vi "UI_List.vi"() -> ()   [LabVIEW 2016]
uses:
  PanelSplitToolkit/QueueManager.llb/Remove.vi
  <vilib>/Utility/error.llb/DialogType.ctl
  PanelSplitToolkit/QueueManager.llb/Valid?.vi
  PanelSplitToolkit/QueueManager.llb/Insert.vi
  PanelSplitToolkit/QueueManager.llb/Destroy.vi
  <vilib>/Platform/TimedLoop/XDataNode/XDataNode.xnode
  <vilib>/Platform/TimedLoop/XDataNode/nitl_modes.ctl
  <vilib>/Platform/TimedLoop/XDataNode/XDNodeRunTimeDep.lvlib
  <vilib>/Platform/TimedLoop/XDataNode/wakeup.ctl
  <vilib>/Platform/TimedLoop/XDataNode/timing_clust.ctl
  SelectPoint2011/SelectPointObj/SelectPointObj.lvclass
  SelectPoint2011/ManualSelectPoint/ManualSelectPoint.lvclass
  <vilib>/Utility/miscctls.llb/LVRowAndColumnTypeDef.ctl
  PanelSplitToolkit/QueueManager.llb/CreatQueue.vi
panel:
  in  "ID":string caption="请输入产品编号:"
  in  "Caller":string
  in  "Pause":bool
  in  "Stop":bool
  in  "手动":bool
  in  "开始":bool
  in  "多列列表框":i32(listbox)
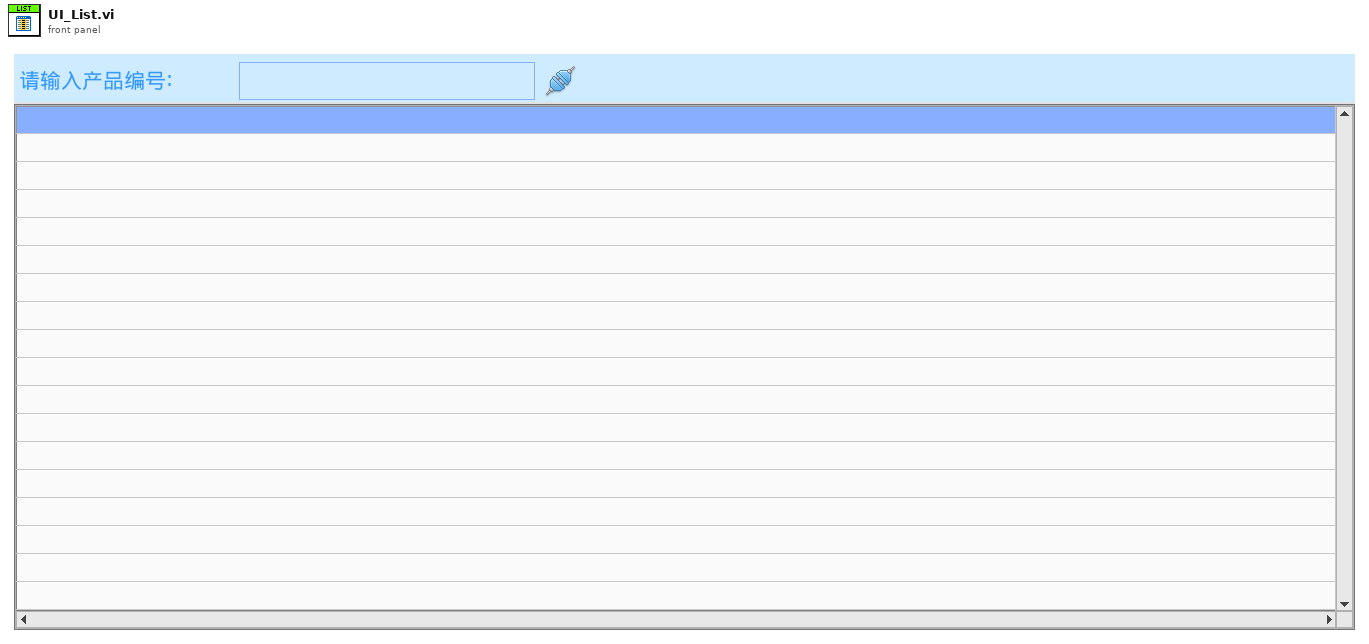
[diagram p1: front panel]
types:
  T1 = cluster{"error":errorcluster, "Event":string, "Data":variant, "Q_Local":string, "SelectPointClass":refnum<class "SelectPointObj.lvclass">, "Q_Caller":string, "ListRef":refnum<vi>}
  T2 = typedef "XDNodeRunTimeDep.lvlib/timing_clust.ctl" = cluster{"Expected End [f-1]":u64, "Actual End [f-1]":u64, "Finished Late? [f-1]":bool, "Expected End [i-1]":u64, "Actual End [i-1]":u64, "Finished Late? [i-1]":bool, "Expected Start [i]":u64, "Actual Start [i]":u64, "Expected Start [f]":u64, "Actual Start [f]":u64, "Source Name":string, "Structure Name":string, "Period":i64, "Deadline":i64, "Offset":i64, "Start":i64, "Priority":i32, "Timeout":i32, "Mode":T3, "Wakeup Reason":T4, "Error":errorcluster, "Source Type":string, "Secondary Source Type":string, "Global End Time":u64, "Global Start Time":u64, "Frame Duration":u64, "Iteration Duration":u64, "Assigned CPU":i32, "I/O Scan Engine Mode":u32}
  T3 = typedef "XDNodeRunTimeDep.lvlib/nitl_modes.ctl" = enum32{"No Change", "Process missed periods, maintain original phase", "Discard missed periods, maintain original phase", "Process missed periods, ignore original phase", "Discard missed periods, ignore original phase"}
  T4 = typedef "XDNodeRunTimeDep.lvlib/wakeup.ctl" = enum32{"Normal", "Aborted", "Asynchronous wakeup", "Timing source error", "Timed loop error", "Timeout"}
  T5 = cluster{"Font Name":string, "Size":u16, "Bold":bool, "Italic":bool, "Underline":bool, "Strikeout":bool, "color":u32}
  T6 = typedef "LVRowAndColumnTypeDef.ctl" = cluster{"Row":i32, "Column":i32}
  T7 = typedef "DialogType.ctl" = u16
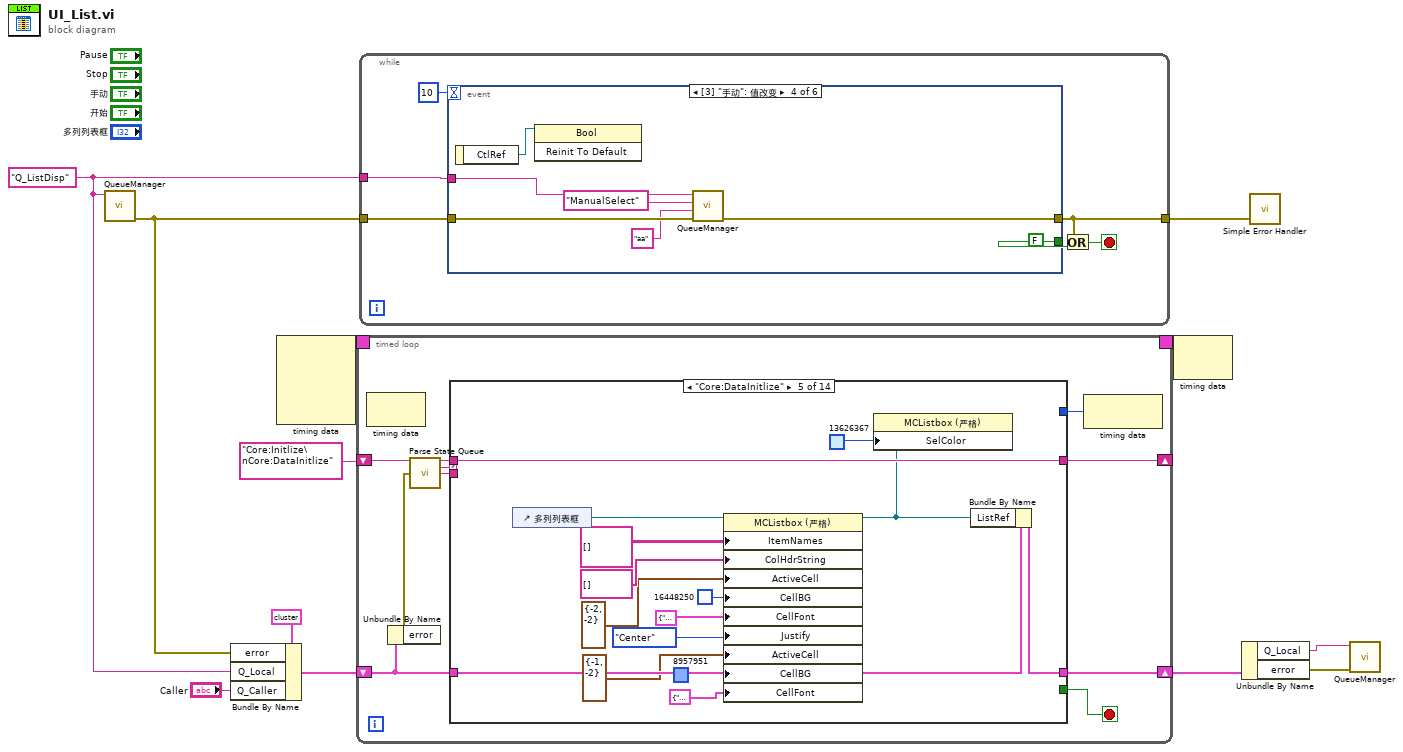
[diagram p0: block diagram]
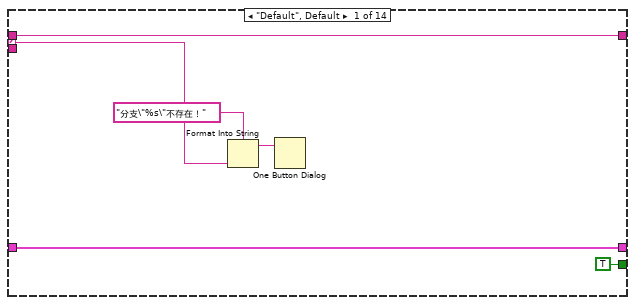
[diagram p2: hidden frame]
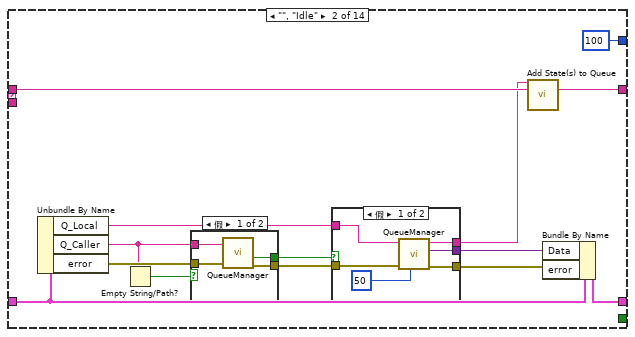
[diagram p3: hidden frame]
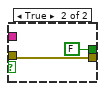
[diagram p4: hidden frame]
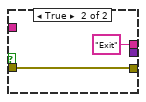
[diagram p5: hidden frame]
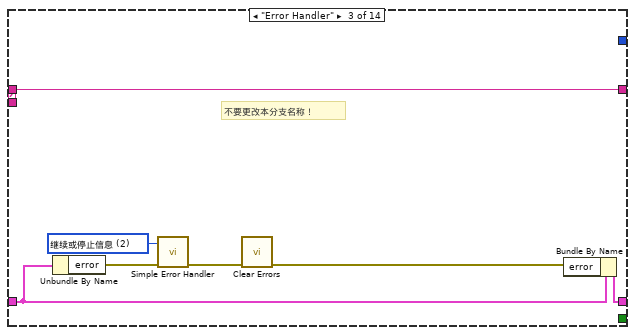
[diagram p6: hidden frame]
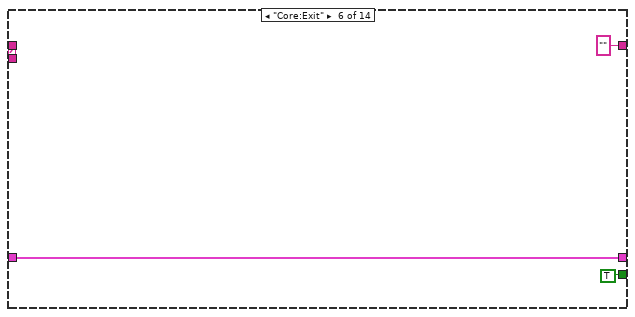
[diagram p8: hidden frame]
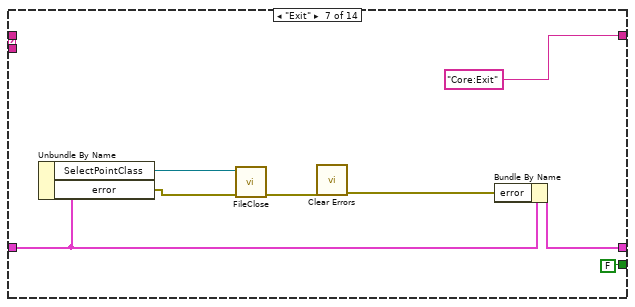
[diagram p9: hidden frame]
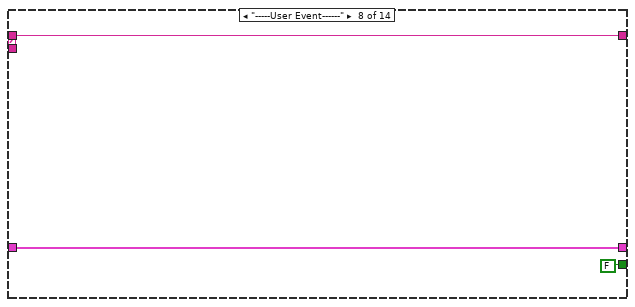
[diagram p10: hidden frame]
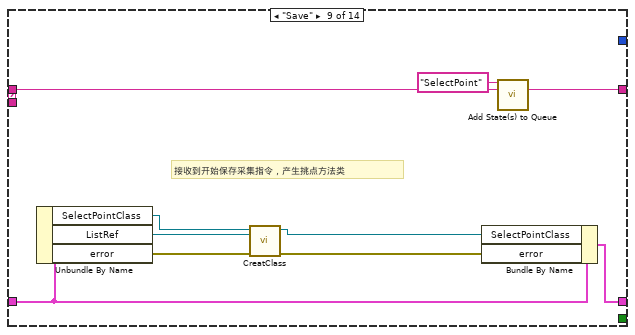
[diagram p11: hidden frame]
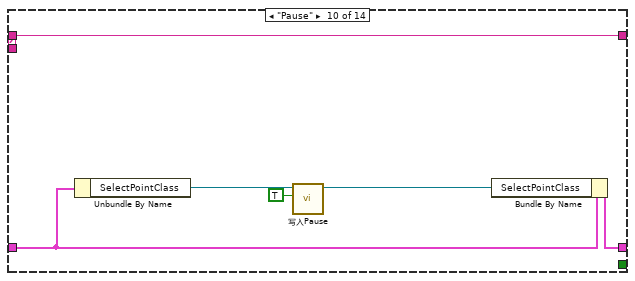
[diagram p12: hidden frame]
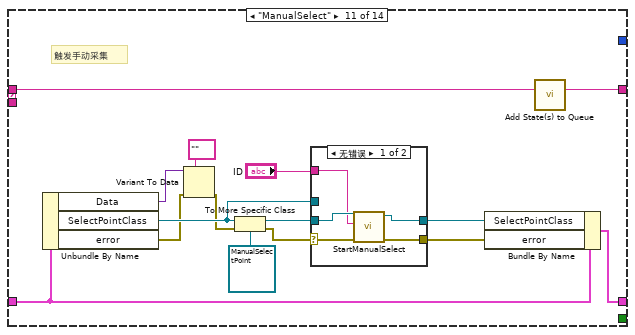
[diagram p13: hidden frame]
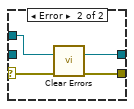
[diagram p14: hidden frame]
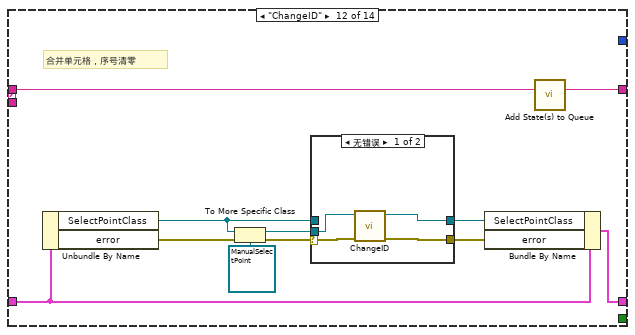
[diagram p15: hidden frame]
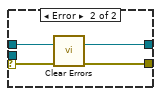
[diagram p16: hidden frame]
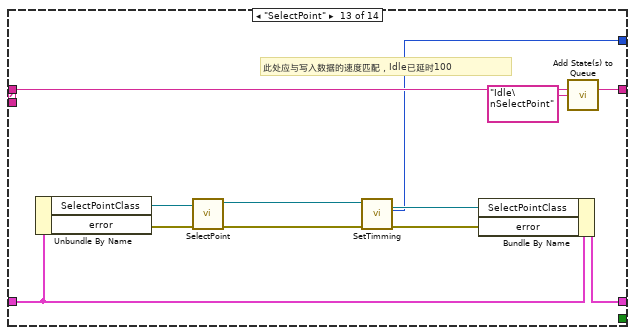
[diagram p17: hidden frame]
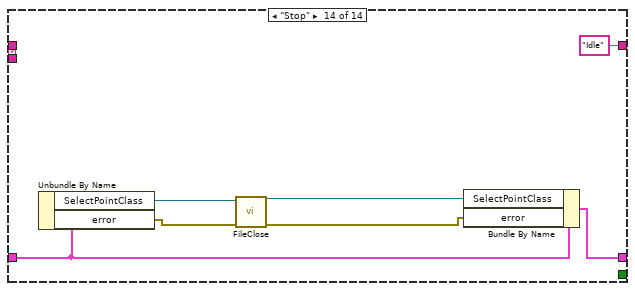
[diagram p18: hidden frame]
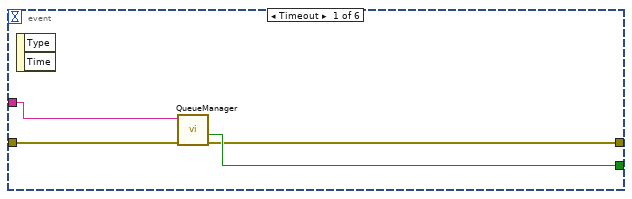
[diagram p19: hidden frame]
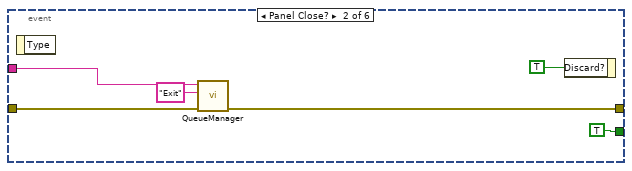
[diagram p20: hidden frame]
diagram:
  w6 = "Q_ListDisp" ("QueueName")
  n1 = call-poly "QueueManager.vi"("QueueName"=w6) -> ("error out"=w4:errorcluster)  [unwired: 9 in, 1 out]
  n2 = Bundle By Name(cluster=T1 {"error"={"status"=FALSE, "code"=0, "source"=""}, "Event"="", "Data"=variant, "Q_Local"="", "SelectPointClass"=refnum, "Q_Caller"="", "ListRef"=refnum} ("TmpData"), "error"=w4, "Q_Local"=w6, "Q_Caller"="Caller") -> (w7:T1)
  n3 = node-c288() -> (w3:T2)  [unwired: 4 in]
  n4 = timed-loop {
    shift-right: [w15] -> w10
    shift-left: w7 -> [w16]
    shift-right: [w14] -> _
    shift-left: "Core:Initlize\nCore:DataInitlize" -> [w22]
    timing: w3 -> [_]
    timing-out: [_] -> w2
    stop <- w18 stop-if-true
    n5 = node-c288() -> ()  [unwired: 1 in, 1 out]
    n6 = Unbundle By Name(w16) -> ("error"=w17:errorcluster)
    n7 = call "Parse State Queue.vi"("State Queue"=w22, "Error In (no error)"=w17) -> ("Remaining States"=w21:string, "Current State"=w20:string, "Arguments"=w19:string)  [unwired: 10 in, 1 out]
    n8 = case shown="\"Core:DataInitlize\"" w20 {
      selector: w20 -> [w30 _ _ _ _ _ _ _ _ _ _ _ _ _]
      tunnel: w21 -> [w31 w43 w67 w69 w84 _ _ w96 w103 w114 w129 w148 w167 _]
      tunnel: w19 -> [_ _ _ _ _ _ _ _ _ _ _ _ _ _]
      tunnel: [TRUE _ _ _ _ TRUE FALSE FALSE _ _ _ _ _ _] -> w18
      tunnel: w16 -> [w32 w42 w63 w68 w83 w86 w91 w97 w106 w110 w127 w146 w165 w171]
      tunnel: [w32 w45 w62 w68 w82 w86 w90 w97 w104 w109 w126 w145 w164 w170] -> w15
      tunnel: [w31 w41 w67 w69 w84 "" ("Remaining States") "Core:Exit" ("Remaining States") w96 w102 w114 w128 w147 w166 "Idle" ("States Out")] -> w14
      tunnel: [_ i64 100 ("周期") _ _ _ _ _ _ _ _ _ _ w162 _] -> w13
      frame "Default", Default {
        n9 = Format Into String(format string="分支\"%s\"不存在！" ("格式字符串"), w30) -> (resulting string=w29:string)  [unwired: 2 in, 1 out]
        n10 = One Button Dialog(message=w29) -> ()  [unwired: 1 in, 1 out]
      }
      frame "", "Idle" {
        n11 = Unbundle By Name(w42) -> ("Q_Local"=w39:string, "Q_Caller"=w35:string, "error"=w38:errorcluster)
        n12 = Empty String/Path?(string/path=w35) -> (empty?=w34:bool)
        n13 = case shown="假" w34 {
          tunnel: w38 -> [w50 w51]
          tunnel: [w49 w51] -> w37
          tunnel: [w48 FALSE ("Not Exist?")] -> w36
          tunnel: w35 -> [w47 _]
          frame False {
            n14 = call-poly "QueueManager.vi"("error in (no error)"=w50, "Queue Name(unamed)"=w47) -> ("error out"=w49:errorcluster, "Not Exist?"=w48:bool)  [unwired: 8 in]
          }
          frame True {
          }
        }
        n15 = case shown="假" w36 {
          tunnel: [w58 w59] -> w46
          tunnel: [w57 _] -> w44
          tunnel: [w56 "Exit" ("Event")] -> w33
          tunnel: w39 -> [w54 _]
          tunnel: w37 -> [w53 w59]
          frame False {
            n16 = call-poly "QueueManager.vi"("Time out(-1)"=50, "error in (no error)"=w53, "Queue Name"=w54) -> ("error out"=w58:errorcluster, "Data"=w57:variant, "Event"=w56:string)  [unwired: 5 in, 1 out]
          }
          frame True {
          }
        }
        n17 = call "Add State(s) to Queue.vi"("State(s) in Front (\"\")"=w33, "State(s) in (\"\")"=w43) -> ("States Out"=w41:string)  [unwired: 13 in]
        n18 = Bundle By Name(cluster=w42, "Data"=w44, "error"=w46) -> (w45:T1)
      }
      frame "Error Handler" {
        w61 = T7 2 items=["无对话框", "确定信息", "继续或停止信息", "确定信息＋警告", "继续/停止+警告"] ("type of dialog (OK msg:1)")
        # "不要更改本分支名称！"
        n19 = Unbundle By Name(w63) -> ("error"=w64:errorcluster)
        n20 = call <vilib>:"Simple Error Handler.vi"("type of dialog (OK msg:1)"=w61, "error in (no error)"=w64) -> ("error out"=w65:errorcluster)  [unwired: 3 in, 4 out]
        n21 = call <vilib>:"Clear Errors.vi"("error in (no error)"=w65) -> ("error out"=w66:errorcluster)  [unwired: 5 in, 1 out]
        n22 = Bundle By Name(cluster=w63, "error"=w66) -> (w62:T1)
      }
      frame "Core:Initlize" {
      }
      frame "Core:DataInitlize" {
        n23 = control-ref of="多列列表框"() -> (w81:refnum<vi>)
        n24 = property class="MCListbox (严格)"(reference=w81, "ItemNames"=string[][] [] ("项名"), "ColHdrString"=string[] [] ("列首字符串[]"), "ActiveCell"=T6 {"Row"=-2, "Column"=-2} ("活动单元格:活动单元格"), "CellBG"=u32 16448250, "CellFont"=T5 {"Font Name"="Tahoma", "Size"=24, "Bold"=FALSE, "Italic"=FALSE, "Underline"=FALSE, "Strikeout"=FALSE, "color"=3381759} ("Active Cell:Cell Font"), "Justify"=enum16{"Left", "Center", "Right"}."Center" ("活动单元格:单元格对齐"), "ActiveCell"=T6 {"Row"=-1, "Column"=-2} ("活动单元格:活动单元格"), "CellBG"=u32 8957951, "CellFont"=T5 {"Font Name"="Tahoma", "Size"=24, "Bold"=FALSE, "Italic"=FALSE, "Underline"=FALSE, "Strikeout"=FALSE, "color"=16448250} ("Active Cell:Cell Font")) -> (reference out=w71:refnum<vi>)  [unwired: 1 in, 1 out]
        n25 = property class="MCListbox (严格)"(reference=w71, "SelColor"=u32 13626367) -> ()  [unwired: 1 in, 2 out]
        n26 = Bundle By Name(cluster=w83, "ListRef"=w71) -> (w82:T1)
      }
      frame "Core:Exit" {
      }
      frame "Exit" {
        n27 = Unbundle By Name(w91) -> ("SelectPointClass"=w93:refnum<class "SelectPointObj.lvclass">, "error"=w92:errorcluster)
        n28 = call-dynamic "FileClose.vi"("error in (no error)"=w92, "SelectPointObj 输入"=w93) -> ("error out"=w89:errorcluster)  [unwired: 8 in, 1 out]
        n29 = call <vilib>:"Clear Errors.vi"("error in (no error)"=w89) -> ("error out"=w88:errorcluster)  [unwired: 5 in, 1 out]
        n30 = Bundle By Name(cluster=w91, "error"=w88) -> (w90:T1)
      }
      frame "-----User Event------" {
      }
      frame "Save" {
        # "接收到开始保存采集指令，产生挑点方法类"
        n31 = Unbundle By Name(w106) -> ("SelectPointClass"=w99:refnum<class "SelectPointObj.lvclass">, "ListRef"=w100:refnum<vi>, "error"=w108:errorcluster)
        n32 = call "CreatClass.vi"("error in"=w108, "ListRef"=w100, "SelectPointObj"=w99) -> ("error out"=w107:errorcluster, "SelectPointObj.lvclass"=w105:refnum<class "SelectPointObj.lvclass">)  [unwired: 7 in]
        n33 = Bundle By Name(cluster=w106, "SelectPointClass"=w105, "error"=w107) -> (w104:T1)
        n34 = call "Add State(s) to Queue.vi"("State(s) in Front (\"\")"="SelectPoint" ("State(s) in Front (\"\")"), "State(s) in (\"\")"=w103) -> ("States Out"=w102:string)  [unwired: 13 in]
      }
      frame "Pause" {
        n35 = Unbundle By Name(w110) -> ("SelectPointClass"=w113:refnum<class "SelectPointObj.lvclass">)
        n36 = call-dynamic "写入Pause.vi"("Pause?"=TRUE, "SelectPointObj输入"=w113) -> ("SelectPointObj输出"=w111:refnum<class "SelectPointObj.lvclass">)  [unwired: 8 in, 1 out]
        n37 = Bundle By Name(cluster=w110, "SelectPointClass"=w111) -> (w109:T1)
      }
      frame "ManualSelect" {
        # "触发手动采集"
        n38 = Unbundle By Name(w127) -> ("Data"=w119:variant, "SelectPointClass"=w120:refnum<class "SelectPointObj.lvclass">, "error"=w118:errorcluster)
        n39 = Variant To Data(error in=w118, type="", Variant=w119) -> (error out=w117:errorcluster)  [unwired: 1 out]
        n40 = To More Specific Class(target class=refnum<class "ManualSelectPoint.lvclass"> refnum ("ManualSelectPoint.lvclass"), reference=w120, error in=w117) -> (specific class reference=w123:refnum<class "ManualSelectPoint.lvclass">, error out=w124:errorcluster)
        n41 = case shown="无错误" w124 {
          selector: w124 -> [w133 w136]
          tunnel: w123 -> [w134 _]
          tunnel: [w132 w135] -> w122
          tunnel: [w131 w137] -> w121
          tunnel: w120 -> [_ w137]
          tunnel: "ID" -> [w130 _]
          frame No Error {
            n42 = call "StartManualSelect.vi"("error in"=w133, "ProductID"=w130, "ManualSelectPoint 输入"=w134) -> ("error out"=w132:errorcluster, "ManualSelectPoint 输出"=w131:refnum<class "ManualSelectPoint.lvclass">)  [unwired: 7 in]
          }
          frame Error {
            n43 = call <vilib>:"Clear Errors.vi"("error in (no error)"=w136) -> ("error out"=w135:errorcluster)  [unwired: 5 in, 1 out]
          }
        }
        n44 = Bundle By Name(cluster=w127, "SelectPointClass"=w121, "error"=w122) -> (w126:T1)
        n45 = call "Add State(s) to Queue.vi"("State(s) in (\"\")"=w129) -> ("States Out"=w128:string)  [unwired: 14 in]
      }
      frame "ChangeID" {
        # "合并单元格，序号清零"
        n46 = Unbundle By Name(w146) -> ("SelectPointClass"=w139:refnum<class "SelectPointObj.lvclass">, "error"=w138:errorcluster)
        n47 = To More Specific Class(target class=refnum<class "ManualSelectPoint.lvclass"> refnum ("ManualSelectPoint.lvclass"), reference=w139, error in=w138) -> (specific class reference=w142:refnum<class "ManualSelectPoint.lvclass">, error out=w143:errorcluster)
        n48 = case shown="无错误" w143 {
          selector: w143 -> [w150 w154]
          tunnel: w142 -> [w152 _]
          tunnel: [w149 w153] -> w141
          tunnel: [w151 w155] -> w140
          tunnel: w139 -> [_ w155]
          frame No Error {
            n49 = call "ChangeID.vi"("error in"=w150, "ManualSelectPoint 输入"=w152) -> ("error out"=w149:errorcluster, "ManualSelectPoint 输出"=w151:refnum<class "ManualSelectPoint.lvclass">)  [unwired: 8 in]
          }
          frame Error {
            n50 = call <vilib>:"Clear Errors.vi"("error in (no error)"=w154) -> ("error out"=w153:errorcluster)  [unwired: 5 in, 1 out]
          }
        }
        n51 = Bundle By Name(cluster=w146, "SelectPointClass"=w140, "error"=w141) -> (w145:T1)
        n52 = call "Add State(s) to Queue.vi"("State(s) in (\"\")"=w148) -> ("States Out"=w147:string)  [unwired: 14 in]
      }
      frame "SelectPoint" {
        # "此处应与写入数据的速度匹配，Idle已延时100"
        n53 = Unbundle By Name(w165) -> ("SelectPointClass"=w159:refnum<class "SelectPointObj.lvclass">, "error"=w158:errorcluster)
        n54 = call-dynamic "SelectPoint.vi"("error in"=w158, "SelectPointObj 输入"=w159) -> ("error out"=w157:errorcluster, "SelectPointObj 输出"=w156:refnum<class "SelectPointObj.lvclass">)  [unwired: 8 in]
        n55 = call-dynamic "SetTimming.vi"("error in (no error)"=w157, "SelectPointObj 输入"=w156) -> ("error out"=w161:errorcluster, "dt"=w162:i64, "SelectPointObj 输出"=w163:refnum<class "SelectPointObj.lvclass">)  [unwired: 7 in]
        n56 = Bundle By Name(cluster=w165, "SelectPointClass"=w163, "error"=w161) -> (w164:T1)
        n57 = call "Add State(s) to Queue.vi"("State(s) in (\"\")"=w167, "State(s) at Back (\"\")"="Idle\nSelectPoint" ("State(s) at Back (\"\")")) -> ("States Out"=w166:string)  [unwired: 13 in]
      }
      frame "Stop" {
        n58 = Unbundle By Name(w171) -> ("SelectPointClass"=w173:refnum<class "SelectPointObj.lvclass">, "error"=w168:errorcluster)
        n59 = call-dynamic "FileClose.vi"("error in (no error)"=w168, "SelectPointObj 输入"=w173) -> ("error out"=w169:errorcluster, "SelectPointObj 输出"=w172:refnum<class "SelectPointObj.lvclass">)  [unwired: 8 in]
        n60 = Bundle By Name(cluster=w171, "SelectPointClass"=w172, "error"=w169) -> (w170:T1)
      }
    }
    n61 = node-c288(w13) -> ()  [unwired: 1 out]
  }
  n62 = while {
    tunnel: w4 -> [w179]
    tunnel: w6 -> [w180]
    tunnel: [w176] -> w9
    stop <- w177 stop-if-true
    n63 = event shown="[3] \"手动\": 值改变" {
      selector: _ -> [_ _ _ _ _ _]
      dyn-events: _ -> [_ _ _ _ _ _]
      timeout: 10 -> [_ _ _ _ _ _]
      tunnel: [w182 TRUE FALSE FALSE FALSE FALSE] -> w178
      tunnel: w180 -> [w184 w189 w195 w202 w208 w214]
      tunnel: w179 -> [w183 w188 w194 w201 w207 w213]
      tunnel: [w181 w187 w193 w200 w206 w212] -> w176
      event Timeout {
        n64 = event-data() -> ()  [unwired: 1 in, 2 out]
        n65 = call-poly "QueueManager.vi"("error in (no error)"=w183, "Queue Name(unamed)"=w184) -> ("error out"=w181:errorcluster, "Not Exist?"=w182:bool)  [unwired: 8 in]
      }
      event Panel Close? {
        n66 = event-data() -> ()  [unwired: 1 in, 1 out]
        n67 = call-poly "QueueManager.vi"("error in"=w188, "Event"="Exit", "QueueName"=w189) -> ("error out"=w187:errorcluster)  [unwired: 7 in, 1 out]
        n68 = event-data("Discard?"=TRUE ("放弃？")) -> ()  [unwired: 1 in, 1 out]
      }
      event "开始": Value Change {
        (unwired) TRUE ("放弃？")
        n69 = event-data() -> ("CtlRef"=w191:refnum<vi>)  [unwired: 1 in]
        n70 = invoke class="Bool" method="Reinit To Default"(reference=w191) -> ()  [unwired: 2 in, 3 out]
        n71 = call-poly "QueueManager.vi"("error in"=w194, "Event"="Save", "QueueName"=w195) -> ("error out"=w193:errorcluster)  [unwired: 7 in, 1 out]
      }
      event "手动": Value Change {
        n72 = event-data() -> ("CtlRef"=w198:refnum<vi>)  [unwired: 1 in]
        n73 = invoke class="Bool" method="Reinit To Default"(reference=w198) -> ()  [unwired: 2 in, 3 out]
        n74 = call-poly "QueueManager.vi"("error in"=w201, "Data"="aa", "Event"="ManualSelect", "QueueName"=w202) -> ("error out"=w200:errorcluster)  [unwired: 6 in, 1 out]
      }
      event "Stop": Value Change {
        (unwired) TRUE ("放弃？")
        n75 = event-data() -> ("CtlRef"=w204:refnum<vi>)  [unwired: 1 in]
        n76 = invoke class="Bool" method="Reinit To Default"(reference=w204) -> ()  [unwired: 2 in, 3 out]
        n77 = call-poly "QueueManager.vi"("error in"=w207, "Event"="Stop", "QueueName"=w208) -> ("error out"=w206:errorcluster)  [unwired: 7 in, 1 out]
      }
      event "Pause": Value Change {
        (unwired) TRUE ("放弃？")
        n78 = event-data() -> ("CtlRef"=w210:refnum<vi>)  [unwired: 1 in]
        n79 = invoke class="Bool" method="Reinit To Default"(reference=w210) -> ()  [unwired: 2 in, 3 out]
        n80 = call-poly "QueueManager.vi"("error in"=w213, "Event"="Pause", "QueueName"=w214) -> ("error out"=w212:errorcluster)  [unwired: 7 in, 1 out]
      }
    }
    n81 = Or(x=w176, y=w178) -> (x .or. y?=w177:bool)
  }
  n82 = node-c288(w2) -> ()  [unwired: 1 out]
  n83 = Unbundle By Name(w10) -> ("Q_Local"=w5:string, "error"=w11:errorcluster)
  n84 = call <vilib>:"Simple Error Handler.vi"("error in (no error)"=w9) -> ()  [unwired: 4 in, 5 out]
  n85 = call-poly "QueueManager.vi"("error in (no error)"=w11, "QueeuName"=w5) -> ()  [unwired: 9 in, 1 out]
